vi "Calc_Moments_PreCalc.vi"(11 "Size":cluster{"X":i32, "Y":i32}) -> (3 "input cluster":cluster{"X2":sgl[], "Y2":sgl[], "XY":sgl[][]})   [LabVIEW 2014]
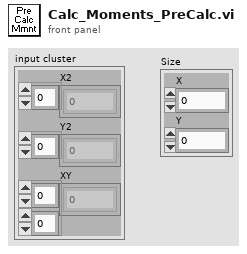
[diagram p1: front panel]
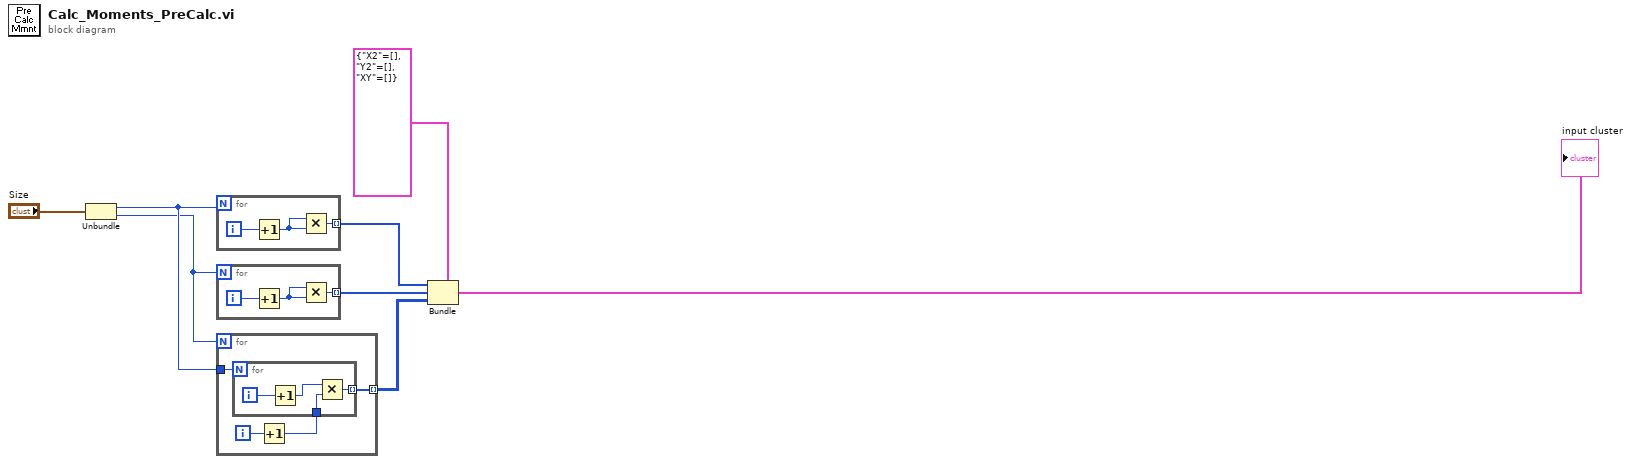
[diagram p0: block diagram]
diagram:
  n1 = Unbundle("Size") -> ("X"=w2:i32, "Y"=w1:i32)
  n2 = for {
    N: w2 -> [_]
    tunnel: [w9] -> w5 mode=indexing
    i -> [w10]
    n3 = Increment(x=w10) -> (x+1=w11:i32)
    n4 = Multiply(x=w11, y=w11) -> (x*y=w9:i32)
  }
  n5 = for {
    N: w1 -> [_]
    tunnel: [w12] -> w6 mode=indexing
    i -> [w13]
    n6 = Increment(x=w13) -> (x+1=w14:i32)
    n7 = Multiply(x=w14, y=w14) -> (x*y=w12:i32)
  }
  n8 = for {
    N: w1 -> [_]
    tunnel: [w16] -> w7 mode=indexing
    tunnel: w2 -> [w15]
    i -> [w18]
    n9 = Increment(x=w18) -> (x+1=w17:i32)
    n10 = for {
      N: w15 -> [_]
      tunnel: [w21] -> w16 mode=indexing
      tunnel: w17 -> [w19]
      i -> [w22]
      n11 = Increment(x=w22) -> (x+1=w20:i32)
      n12 = Multiply(x=w20, y=w19) -> (x*y=w21:i32)
    }
  }
  n13 = Bundle(cluster=cluster{"X2":sgl[], "Y2":sgl[], "XY":sgl[][]} {"X2"=[], "Y2"=[], "XY"=[]} ("input cluster"), "X2"=w5, "Y2"=w6, "XY"=w7) -> (→"input cluster":cluster{"X2":sgl[], "Y2":sgl[], "XY":sgl[][]})
